vi "Add content to Engine library.vi"(6 "Project Name":string, 8 "error in":errorcluster, 9 "Project Root":path, 10 "CD Wizard - Internal Data":T1, 11 "Inline-Async":refnum<class "NIVS_Inline HW Interface (Inline-Async).lvclass">) -> (0 "error out":errorcluster)   [LabVIEW 2020, in "NIVS_Inline HW Interface (Inline-Async).lvclass"]
doc: "Add all virtual folders and VIs to the Engine library."
uses:
  NIVS_Inline HW Interface (Inline-Async).lvclass
  NIVS_Consolidated_CDW_MetaDataObj/Internal data.ctl
  C:/dev/Karthick/FPGA Addons Packages/niveristand-custom-device-wizard/ProjectTemplate/Source/NI VeriStand/Custom Device/Template Classes/NIVS_CD Template/NIVS_CD Template.lvclass
  NIVS_Consolidated_CDW_MetaDataObj/CD Engine lvlib.ctl
  NIVS_Consolidated_CDW_MetaDataObj/Add Item - Type.ctl
  NIVS_CD Template/NIVS_CD Template.lvclass/NIVS_CD Template.ctl
  NIVS_Consolidated_CDW_MetaDataObj/CD Engine lvlib.vi
  NIVS_Consolidated_CDW_MetaDataObj/NIVS_Consolidated_CDW_MetaDataObj.lvclass
  NIVS_CD Template/NIVS_CD Template.lvclass
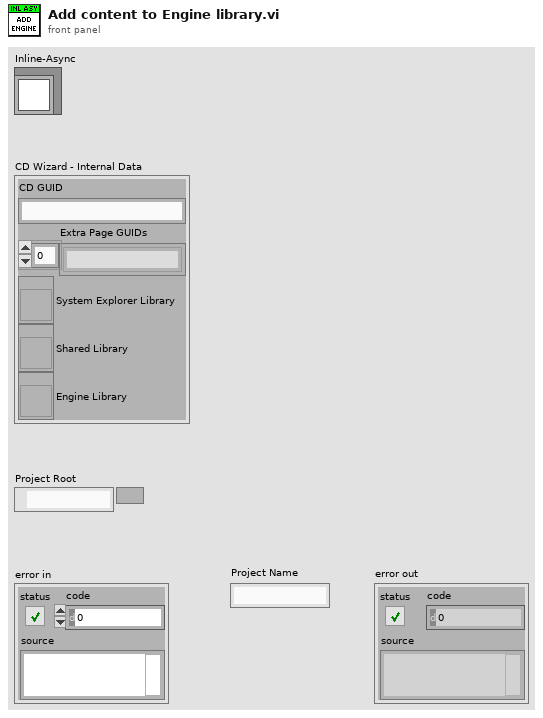
[diagram p1: front panel]
types:
  T1 = typedef "NIVS_Consolidated_CDW_MetaDataObj.lvclass/Internal data.ctl" = cluster{"CD GUID":string, "Extra Page GUIDs":string[], "System Explorer Library":refnum<vi>, "Shared Library":refnum<vi>, "Engine Library":refnum<vi>}
  T2 = typedef "NIVS_Consolidated_CDW_MetaDataObj.lvclass/CD Engine lvlib.ctl" = enum16{"LibraryFileName", "LibraryFolderName", "Engine.FolderName", "Engine.Init.FolderName", "Engine.Run.FolderName", "Engine.Shutdown.FolderName", "Types.FolderName", "Engine.RT Driver VI.TemplatePath", "Engine.RT Driver VI.FileName", "Engine.PPL.RT Driver VI_InlineAsync.FileName", "Engine.RTStateVariables.Name", "Engine.PPL.RTStateVariables.Name", "Engine.RTStateVariables.Name.NoExtension", "Engine.Async.NameExtension", "Engine.Async.TemplateName", "Engine.PPL.Async.TemplateName", "Engine.PPL.Async.InitVSGlobals.Name", "Engine.PPL.RT Driver VI_Inline.FileName", "Engine.LaunchCommandLoop.Name", "Engine.CommandLoop.Name"}
  T3 = typedef "NIVS_Consolidated_CDW_MetaDataObj.lvclass/Add Item - Type.ctl" = string
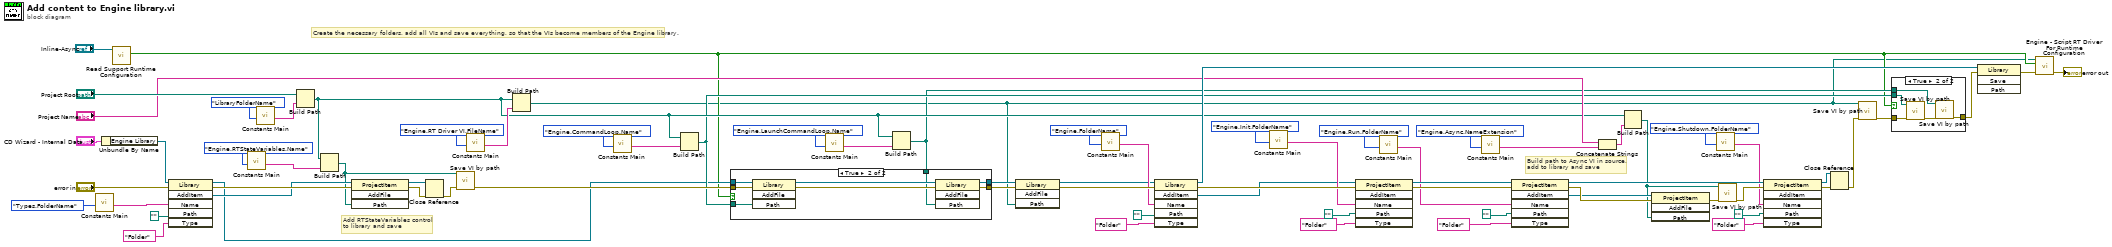
[diagram p0: block diagram]
diagram:
  # "Create the necessary folders, add all VIs and save everything, so that the VIs become members of the Engine library."
  # "Add RTStateVariables control\nto library and save"
  # "Build path to Async VI in source,\nadd to library and save"
  n1 = call-poly "Constants Main.vi"("Action"=CD_Engine_lvlib."Types.FolderName") -> ("Output"=w54:string)  [unwired: 10 in]
  n2 = Unbundle By Name("CD Wizard - Internal Data") -> ("Engine Library"=w44:refnum<vi>)
  n3 = call "Read Support Runtime Configuration.vi"("NIVS_CD Template in"="Inline-Async") -> ("Support Runtime Configuration"=w2:bool)  [unwired: 8 in, 2 out]
  n4 = invoke class="Library" method="AddItem"(reference=w44, error in="error in", "Name"=w54, "Path"=path "", "Type"=T3 "Folder" ("Add Item - Type")) -> (reference out=w5:refnum<vi>, error out=w68:errorcluster, "AddItem"=w25:refnum<vi>)  [unwired: 1 in, 3 out]
  n5 = call-poly "Constants Main.vi"("Action"=CD_Engine_lvlib."Engine.RTStateVariables.Name") -> ("Output"=w17:string)  [unwired: 10 in]
  n6 = call-poly "Constants Main.vi"("Action"=CD_Engine_lvlib."LibraryFolderName") -> ("Output"=w46:string)  [unwired: 10 in]
  n7 = Build Path(base path="Project Root", name or relative path=w46) -> (appended path=w8:path)
  n8 = Build Path(base path=w8, name or relative path=w17) -> (appended path=w24:path)
  n9 = invoke class="ProjectItem" method="AddFile"(reference=w25, error in=w68, "Path"=w24) -> (reference out=w15:refnum<vi>, error out=w72:errorcluster)  [unwired: 1 in, 2 out]
  n10 = Close Reference(reference=w15, error in (no error)=w72) -> (error out=w66:errorcluster)
  n11 = call "Save VI by path.vi"("error in (no error)"=w66, "VI path"=w24) -> ("error out"=w67:errorcluster)  [unwired: 9 in]
  n12 = call-poly "Constants Main.vi"("Action"=CD_Engine_lvlib."Engine.RT Driver VI.FileName") -> ("Output"=w48:string)  [unwired: 10 in]
  n13 = Build Path(base path=w8, name or relative path=w48) -> (appended path=w1:path)
  n14 = call-poly "Constants Main.vi"("Action"=CD_Engine_lvlib."Engine.CommandLoop.Name") -> ("Output"=w11:string)  [unwired: 10 in]
  n15 = Build Path(base path=w8, name or relative path=w11) -> (appended path=w7:path)
  n16 = call-poly "Constants Main.vi"("Action"=CD_Engine_lvlib."Engine.LaunchCommandLoop.Name") -> ("Output"=w10:string)  [unwired: 10 in]
  n17 = Build Path(base path=w8, name or relative path=w10) -> (appended path=w6:path)
  n18 = case shown="True" w2 {
    tunnel: w5 -> [w75 w81]
    tunnel: w67 -> [w76 w84]
    tunnel: w7 -> [_ w80]
    tunnel: w6 -> [_ w78]
    tunnel: [w75 w77] -> w4
    tunnel: [w76 w82] -> w60
    frame False {
    }
    frame True {
      n19 = invoke class="Library" method="AddFile"(reference=w81, error in=w84, "Path"=w80) -> (reference out=w79:refnum<vi>, error out=w83:errorcluster)  [unwired: 1 in, 2 out]
      n20 = invoke class="Library" method="AddFile"(reference=w79, error in=w83, "Path"=w78) -> (reference out=w77:refnum<vi>, error out=w82:errorcluster)  [unwired: 1 in, 2 out]
    }
  }
  n21 = invoke class="Library" method="AddFile"(reference=w4, error in=w60, "Path"=w1) -> (reference out=w3:refnum<vi>, error out=w59:errorcluster)  [unwired: 1 in, 2 out]
  n22 = call-poly "Constants Main.vi"("Action"=CD_Engine_lvlib."Engine.FolderName") -> ("Output"=w41:string)  [unwired: 10 in]
  n23 = invoke class="Library" method="AddItem"(reference=w3, error in=w59, "Name"=w41, "Path"=path "", "Type"=T3 "Folder" ("Add Item - Type")) -> (reference out=w28:refnum<vi>, error out=w65:errorcluster, "AddItem"=w39:refnum<vi>)  [unwired: 1 in, 3 out]
  n24 = call-poly "Constants Main.vi"("Action"=CD_Engine_lvlib."Engine.Init.FolderName") -> ("Output"=w50:string)  [unwired: 10 in]
  n25 = invoke class="ProjectItem" method="AddItem"(reference=w39, error in=w65, "Name"=w50, "Path"=path "", "Type"=T3 "Folder" ("Add Item - Type")) -> (reference out=w37:refnum<vi>, error out=w64:errorcluster)  [unwired: 1 in, 4 out]
  n26 = call-poly "Constants Main.vi"("Action"=CD_Engine_lvlib."Engine.Run.FolderName") -> ("Output"=w35:string)  [unwired: 10 in]
  n27 = call-poly "Constants Main.vi"("Action"=CD_Engine_lvlib."Engine.Async.NameExtension") -> ("Output"=w19:string)  [unwired: 10 in]
  n28 = invoke class="ProjectItem" method="AddItem"(reference=w37, error in=w64, "Name"=w35, "Path"=path "", "Type"=T3 "Folder" ("Add Item - Type")) -> (reference out=w29:refnum<vi>, error out=w71:errorcluster, "AddItem"=w23:refnum<vi>)  [unwired: 1 in, 3 out]
  n29 = Concatenate Strings("Project Name", w19) -> (w22:string)
  n30 = Build Path(base path=w8, name or relative path=w22) -> (appended path=w21:path)
  n31 = invoke class="ProjectItem" method="AddFile"(reference=w23, error in=w71, "Path"=w21) -> (error out=w70:errorcluster)  [unwired: 1 in, 3 out]
  n32 = call-poly "Constants Main.vi"("Action"=CD_Engine_lvlib."Engine.Shutdown.FolderName") -> ("Output"=w27:string)  [unwired: 10 in]
  n33 = call "Save VI by path.vi"("error in (no error)"=w70, "VI path"=w21) -> ("error out"=w63:errorcluster)  [unwired: 9 in]
  n34 = invoke class="ProjectItem" method="AddItem"(reference=w29, error in=w63, "Name"=w27, "Path"=path "", "Type"=T3 "Folder" ("Add Item - Type")) -> (reference out=w26:refnum<vi>, error out=w74:errorcluster)  [unwired: 1 in, 4 out]
  n35 = Close Reference(reference=w26, error in (no error)=w74) -> (error out=w73:errorcluster)
  n36 = call "Save VI by path.vi"("error in (no error)"=w73, "VI path"=w1) -> ("error out"=w62:errorcluster)  [unwired: 9 in]
  n37 = case shown="True" w2 {
    tunnel: w62 -> [w85 w90]
    tunnel: [w85 w88] -> w61
    tunnel: w7 -> [_ w87]
    tunnel: w6 -> [_ w86]
    frame False {
    }
    frame True {
      n38 = call "Save VI by path.vi"("error in (no error)"=w90, "VI path"=w87) -> ("error out"=w89:errorcluster)  [unwired: 9 in]
      n39 = call "Save VI by path.vi"("error in (no error)"=w89, "VI path"=w86) -> ("error out"=w88:errorcluster)  [unwired: 9 in]
    }
  }
  n40 = invoke class="Library" method="Save"(reference=w28, error in=w61) -> (error out=w58:errorcluster)  [unwired: 2 in, 3 out]
  n41 = call "Engine - Script RT Driver For Runtime Configuration.vi"("error in"=w58, "Support Runtime Configuration"=w2, "RT Driver VI Path"=w1) -> ("error out"=→"error out":errorcluster)  [unwired: 8 in]
